vi "WBRT Derivative.vi"(8 "dt":dbl, 11 "Variable":dbl) -> (3 "Derivative":dbl)   [LabVIEW 2012]
doc: "Simple derivative function.\n\nAuthor: Brandon Steele\n\nCopyright: Brigham Young University"
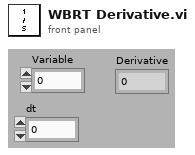
[diagram p1: front panel]
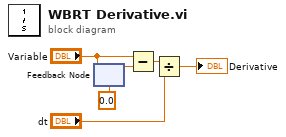
[diagram p0: block diagram]
diagram:
  n1 = feedback-in #1("Variable") -> ()
  n2 = feedback #1(0.0 ("Variable")) -> (w4:dbl)
  n3 = Subtract(x="Variable", y=w4) -> (x-y=w3:dbl)
  n4 = Divide(x=w3, y="dt") -> (x/y=→"Derivative":dbl)
